vi "Parse-Create_New_Line.vi"(7 "Interval":i32=3, 10 "Existing Row":T1[](array[typedef])) -> (2 "New Row":T1[](array[typedef]))   [LabVIEW 2020]
doc: "<B>Description:</B> Generates a array of Tiles. The first element is a Wall, and then every <Interval> is a Wall.\n\n<B>Date:</B> 05/2019\n<B>Author:</B> Luke Jarocki, Choose Movement Consulting, LLC"
uses:
  Controls/TileColor.ctl
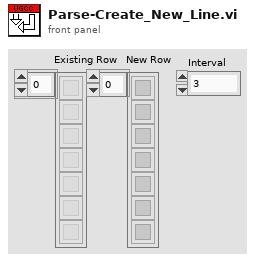
[diagram p1: front panel]
types:
  T1 = typedef "TileColor.ctl" = u16
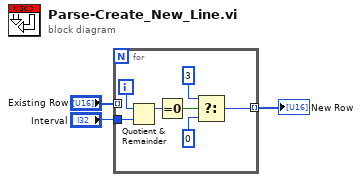
[diagram p0: block diagram]
diagram:
  n1 = for {
    tunnel: "Existing Row" -> [_] mode=indexing
    tunnel: [w7] -> w2 mode=indexing
    tunnel: "Interval" -> [w4]
    i -> [w10]
    n2 = Quotient & Remainder(x=w10, y=w4) -> (x-y*floor(x/y)=w9:i32)  [unwired: 1 out]
    n3 = Equal To 0?(x=w9) -> (x = 0?=w8:bool)
    n4 = Select(t=T1 3 ("Tile"), s=w8, f=T1 0 ("Tile")) -> (s? t:f=w7:T1)
  }
  "New Row" <- w2
